vi "Convert R to T - DBL Array.vi"(8 "error in":errorcluster, 9 "R (kO)":dbl[](array[numeric])=[3.893, 10.0, 29.49], 10 "Tref (C)":dbl[](array[numeric])=[50.0, 25.0, 0.0], 11 "R":dbl[](array[numeric]) caption="R (kOhm)") -> (0 "error out":errorcluster, 3 "T":dbl[](array[numeric]) caption="T (degC)")   [LabVIEW 2015, in "Temperature.lvlib"]
doc: "Converts an array of thermistor resistance in kOhms to an array of temperature a temperature in degrees Celsius"
uses:
  Temperature.lvlib
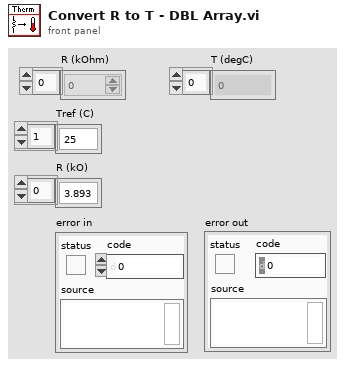
[diagram p1: front panel]
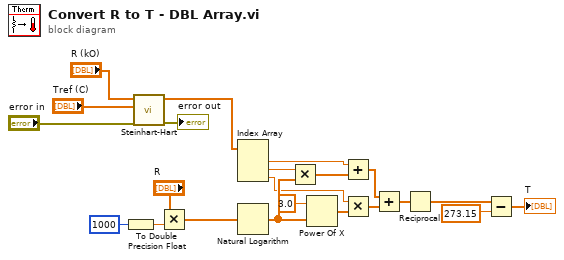
[diagram p0: block diagram]
diagram:
  n1 = To Double Precision Float(number=1000) -> (double precision float=w1:dbl)
  n2 = call "Steinhart-Hart.vi"("error in"="error in", "Tref (C)"="Tref (C)", "R (kO)"="R (kO)") -> ("error out"=→"error out":errorcluster, "Coefficients"=w22:dbl[])  [unwired: 7 in]
  n3 = Multiply(x="R", y=w1) -> (x*y=w7:dbl[])
  n4 = Index Array(array=w22) -> (element #1=w21:dbl, element #2=w19:dbl, element #3=w16:dbl)  [unwired: 3 in]
  n5 = Natural Logarithm(1:w7) -> (0:w18:dbl[])
  n6 = Multiply(x=w19, y=w18) -> (x*y=w17:dbl[])
  n7 = Power Of X(1:w18, 2:3.0 ("y")) -> (0:w15:dbl[])
  n8 = Add(x=w21, y=w17) -> (x+y=w13:dbl[])
  n9 = Multiply(x=w16, y=w15) -> (x*y=w14:dbl[])
  n10 = Add(x=w13, y=w14) -> (x+y=w12:dbl[])
  n11 = Reciprocal(x=w12) -> (1/x=w11:dbl[])
  n12 = Subtract(x=w11, y=273.15) -> (x-y=→"T":dbl[])
